vi "REx - Send Command.vi"(0 "Remote Connection Handle in":T2, 7 "Command Data Element in":T1, 11 "error in (no error)":errorcluster) -> (4 "Remote Connection Handle out":T2, 8 "Command Data Element out":T1, 15 "error out":errorcluster)   [LabVIEW 2012, in "Beta Cmd.lvclass"]
uses:
  Beta Cmd.lvclass
  _REx/Components/Remote Connection Session/Typedefs/Session Handle.ctl
  _REx/Components/Remote Connection Session/Remote Connection Session.lvclass
  STYP - Command Data Element.ctl
  set Command Data Element.vi
  get Command Data Element.vi
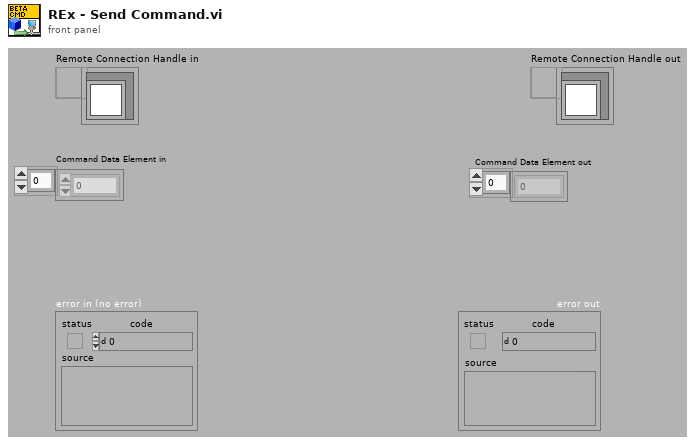
[diagram p1: front panel]
types:
  T1 = typedef "Beta Cmd.lvclass/STYP - Command Data Element.ctl" = dbl[]
  T2 = typedef "REx.lvlib/Remote Connection Session.lvclass/Session Handle.ctl" = refnum<data-value>
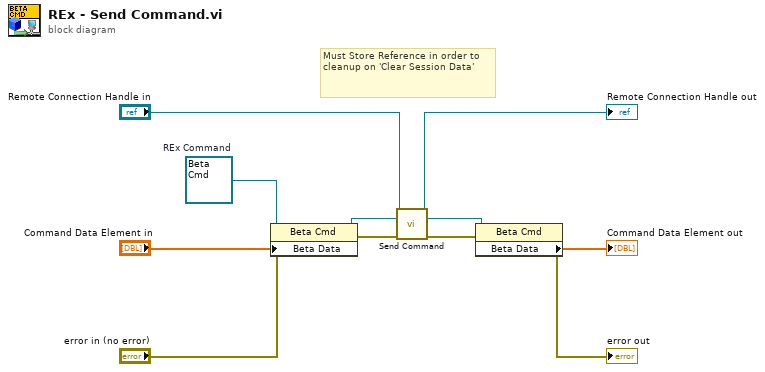
[diagram p0: block diagram]
diagram:
  w5 = refnum<class "Beta Cmd.lvclass"> refnum  # REx Command
  # "Must Store Reference in order to cleanup on 'Clear Session Data'"
  n1 = property class="Beta Cmd"(reference=w5, error in="error in (no error)", "Beta Data"="Command Data Element in") -> (reference out=w3:refnum<class "Beta Cmd.lvclass">, error out=w7:errorcluster)
  n2 = call "Send Command.vi"("Session Handle in"="Remote Connection Handle in", "REx Command in"=w3, "error in (no error)"=w7) -> ("Session Handle out"=→"Remote Connection Handle out":T2, "REx Command out"=w2:refnum<class "Beta Cmd.lvclass">, "error out"=w6:errorcluster)  [unwired: 10 in]
  n3 = property class="Beta Cmd"(reference=w2, error in=w6) -> (error out=→"error out":errorcluster, "Beta Data"=→"Command Data Element out":T1)  [unwired: 1 out]
